vi "SetPayloadDVR.vi"(11 "PayloadDVR":refnum<data-value>) -> (5 "Msg":refnum<class "Msg.lvclass">)   [LabVIEW 2020, in "_Template.lvlib" / "{{Msg}}.lvlib" / "Msg.lvclass"]
uses:
  Msg.lvclass
  Payload.ctl
  Msg.lvclass/Msg.ctl
  {{Msg}}.lvlib
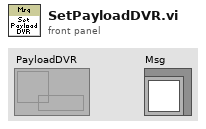
[diagram p1: front panel]
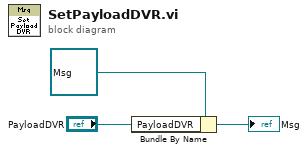
[diagram p0: block diagram]
diagram:
  n1 = Bundle By Name(cluster=refnum<class "Msg.lvclass"> refnum ("Msg"), "PayloadDVR"="PayloadDVR") -> (→"Msg":refnum<class "Msg.lvclass">)
